vi "getFPimage1.vi"(7 "LabVIEW Web Service Request":refnum<class "Web Request.lvclass">) -> ()   [LabVIEW 2014]
uses:
  <vilib>/wsapi/Web Request.lvclass
panel:
  # "Use the Web Service Request input terminal to call the VIs on the Web Services palette. Do not remove it from the connector pane unless you don't need access to the palette."
  # "Each additional control wired to the connector pane will be available as an input in the URL. To include an indicator in terminal-mode output (the default setting), it must also be wired to the connector pane."
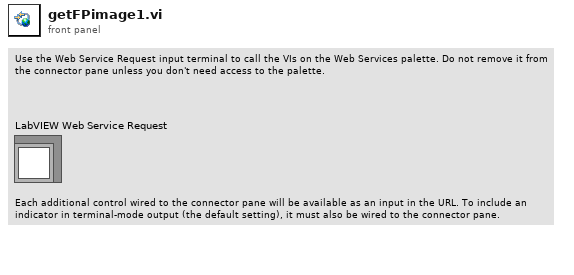
[diagram p1: front panel]
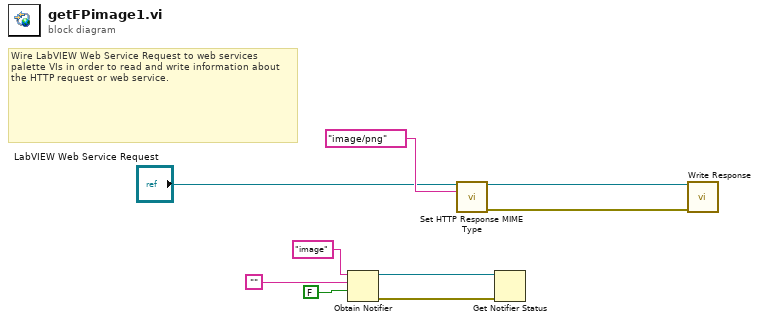
[diagram p0: block diagram]
diagram:
  # "Wire LabVIEW Web Service Request to web services palette VIs in order to read and write information about the HTTP request or web service."
  n1 = Obtain Notifier(name (unnamed)="image", notification data type="", create if not found? (T)=FALSE) -> (notifier out=w7:refnum<notifier>, error out=w6:errorcluster)  [unwired: 1 in, 1 out]
  n2 = call <vilib>:"Set HTTP Response MIME Type.vi"("LabVIEW Web Service Request"="LabVIEW Web Service Request", "MIME type (text/html)"="image/png") -> ("LabVIEW Web Service Request out"=w3:refnum<class "Web Request.lvclass">, "error out"=w2:errorcluster)  [unwired: 12 in]
  n3 = Get Notifier Status(notifier=w7, error in (no error)=w6) -> ()  [unwired: 5 out]
  n4 = call <vilib>:"Write Response.vi"("LabVIEW Web Service Request"=w3, "error in (no error)"=w2) -> ()  [unwired: 12 in, 2 out]
